vi "TilesLoop.vi"(8 "error in (no error)":errorcluster, 11 "Engine in":refnum<class "Engine.lvclass">) -> (0 "error out":errorcluster)   [LabVIEW 2019, in "RT_Game.lvlib" / "Engine.lvclass"]
uses:
  Engine.lvclass
  TilesLoopData.ctl
  Game/Coordinate.ctl
  Game/SlideJob.ctl
  Game/ScreenSide.ctl
  Engine.lvclass/Engine.ctl
  SetTilesData.ctl
  SetTileData.ctl
  MessageCluster.ctl
  <vilib>/Utility/error.llb/Error Cluster From Error Code.vi
  <vilib>/rvi/errors/niLvFpgaAdjustHostInterfaceError.vi
  Globals.vi
  <vilib>/rvi/interface/nirviMethod/nirviMethod.xnode
  FPGA_Interface.ctl
  FPGA Bitfiles/myriogameconsole_FPGATarget_Main_ntsPRcBZGxk.lvbitx
  Game/Game.lvclass
  <vilib>/FPGAPlugInAG/myRIO-1900/niLvFpga_WriteFifo_myRIO-1900.vi
  <vilib>/rvi/errors/niLvFpgaMergeErrorWithErrorCode.vi
  RT_Game.lvlib
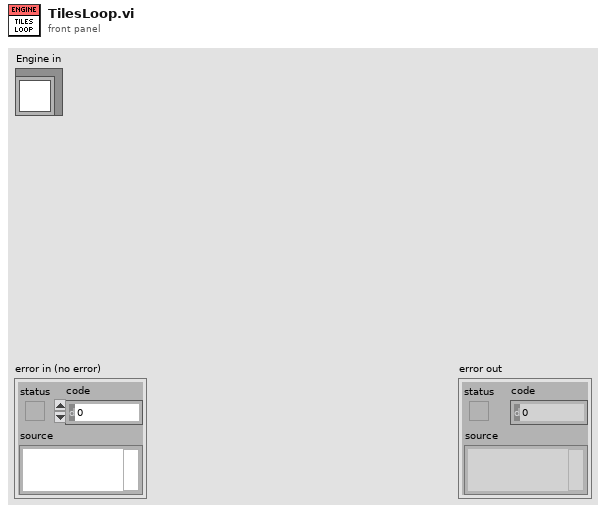
[diagram p1: front panel]
types:
  T1 = typedef "RT_Game.lvlib/Engine.lvclass/TilesLoopData.ctl" = cluster{"TilesToDraw":u64[], "CameraPos":T2, "MoveDistance":T2, "LeftRightBuffer":T3[], "leftrightBufferSize":i16, "leftrightBufferCount":i16, "slidespeed_x":dbl, "delta_t":dbl, "Moving?":bool, "UpDownBuffer":T3[], "updownBufferSize":i16, "updownBufferCount":i16, "slidespeed_y":dbl}
  T2 = typedef "RT_Game.lvlib/Game.lvclass/Coordinate.ctl" = cluster{"x":dbl, "y":dbl}
  T3 = typedef "RT_Game.lvlib/Engine.lvclass/SlideJob.ctl" = cluster{"Pixel":u32[], "Side":T4}
  T4 = typedef "RT_Game.lvlib/Game.lvclass/ScreenSide.ctl" = enum16{"up", "down", "left", "right", "none"}
  T5 = typedef "RT_Game.lvlib/Engine.lvclass/SetTilesData.ctl" = cluster{"TileCodes":u32[][], "Position":T2}
  T6 = typedef "RT_Game.lvlib/Engine.lvclass/SetTileData.ctl" = cluster{"TileCode":u32, "Position":T2}
  T7 = typedef "RT_Game.lvlib/Engine.lvclass/MessageCluster.ctl" = cluster{"Message":string, "Data":variant}
  T8 = typedef "FPGA_Interface.ctl" = refnum<k20>
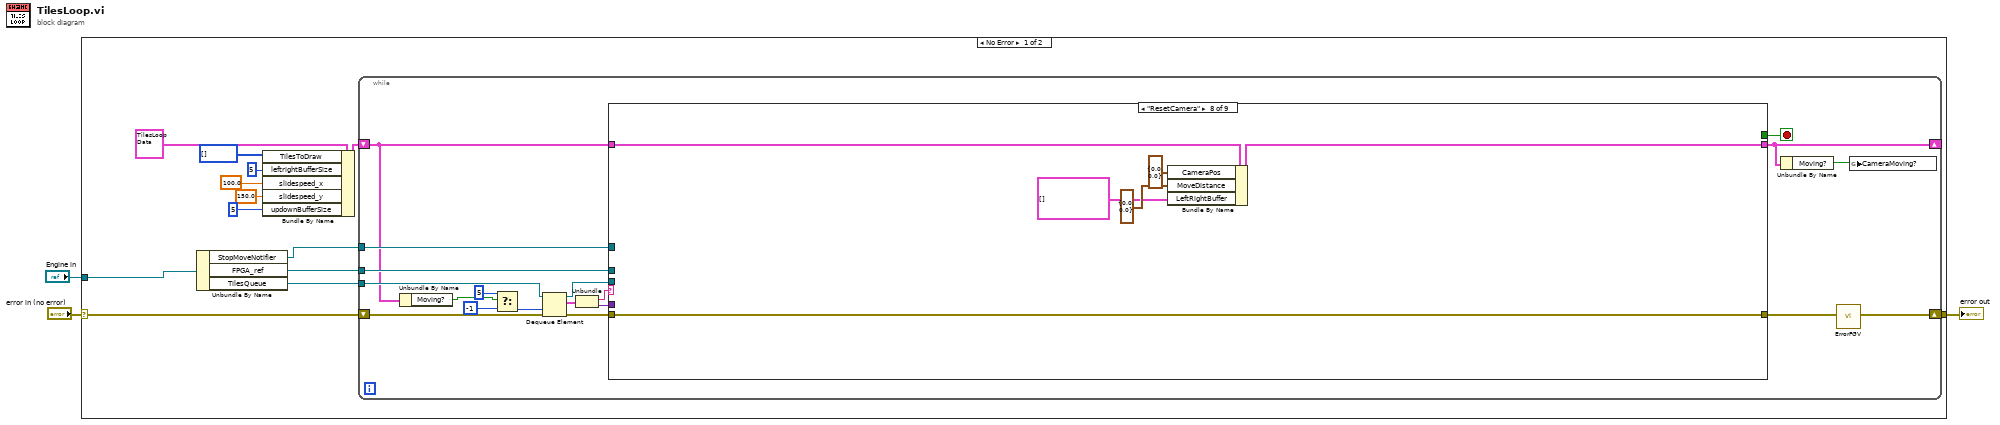
[diagram p0: block diagram]
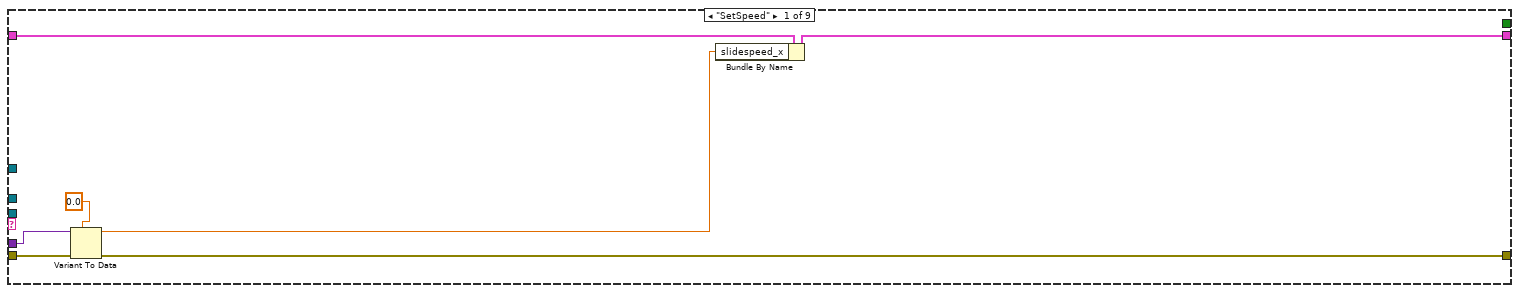
[diagram p2: hidden frame]
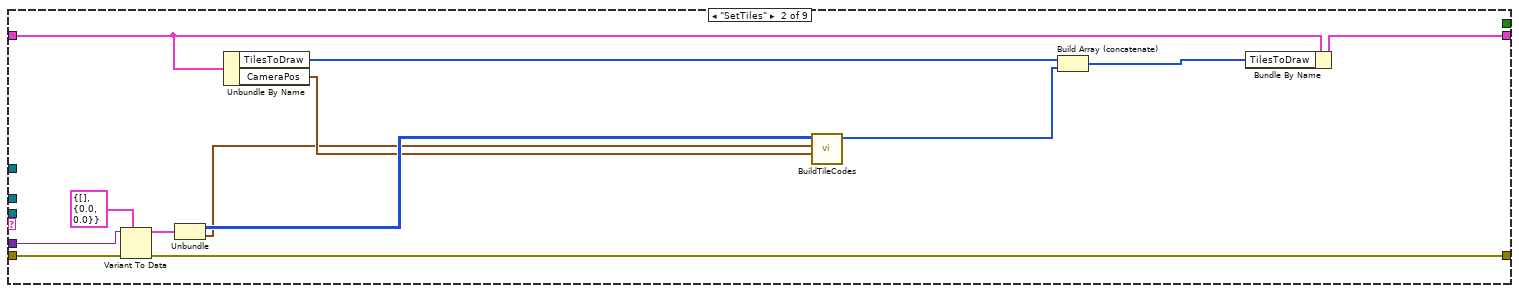
[diagram p3: hidden frame]
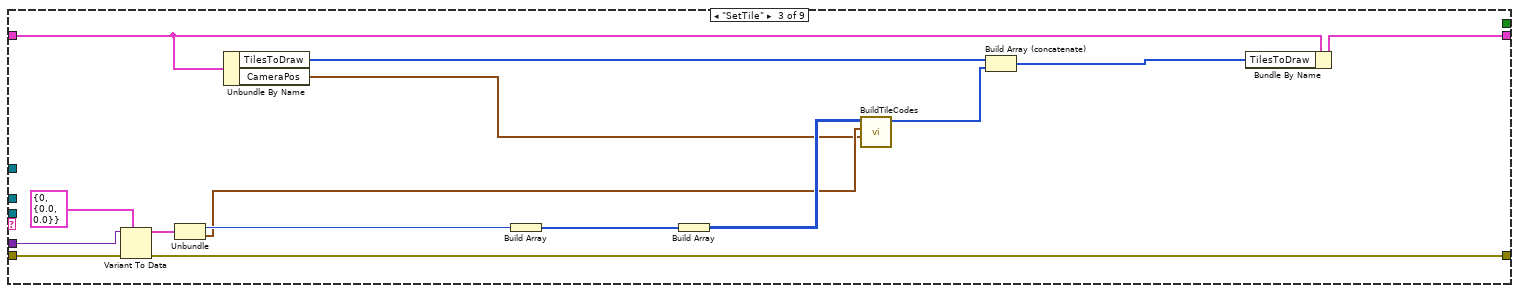
[diagram p4: hidden frame]
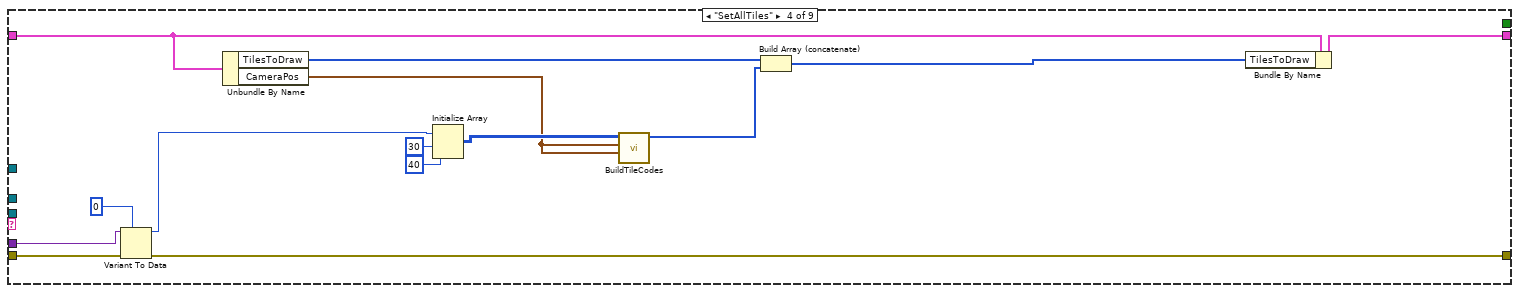
[diagram p5: hidden frame]
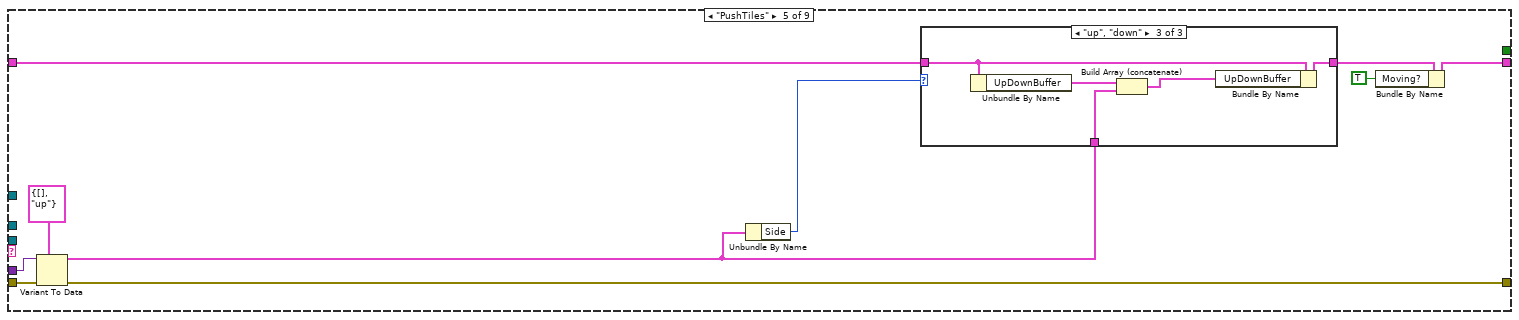
[diagram p6: hidden frame]
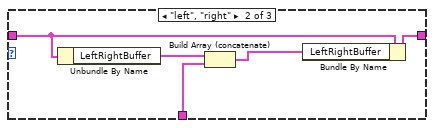
[diagram p8: hidden frame]
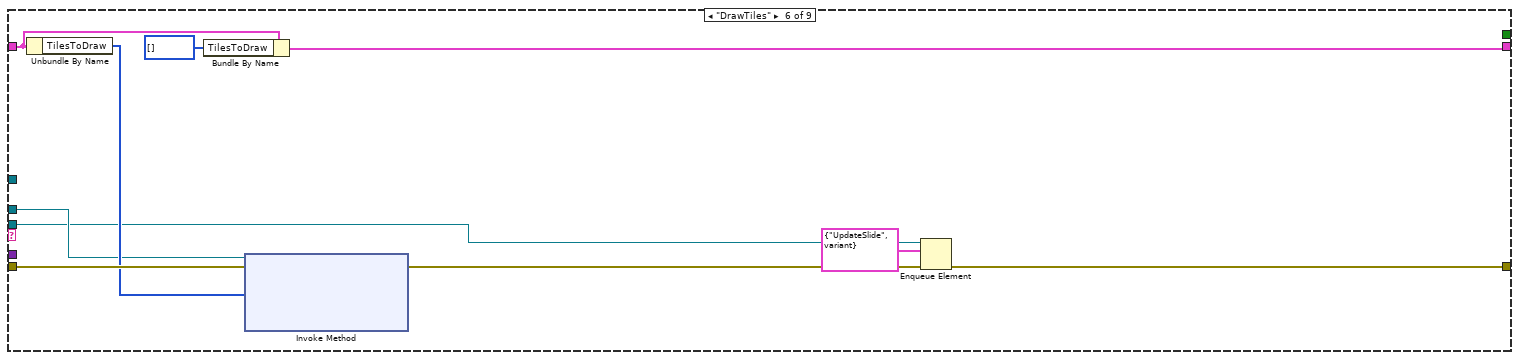
[diagram p9: hidden frame]
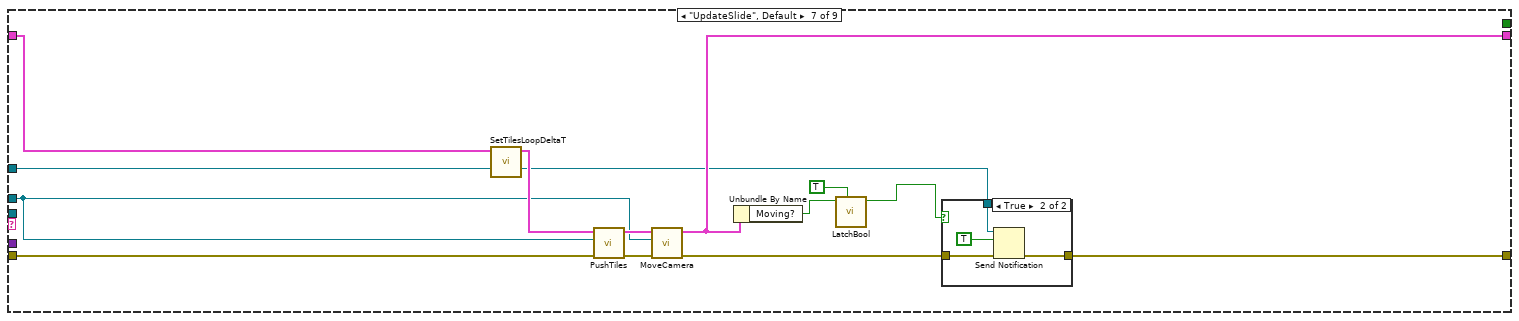
[diagram p10: hidden frame]
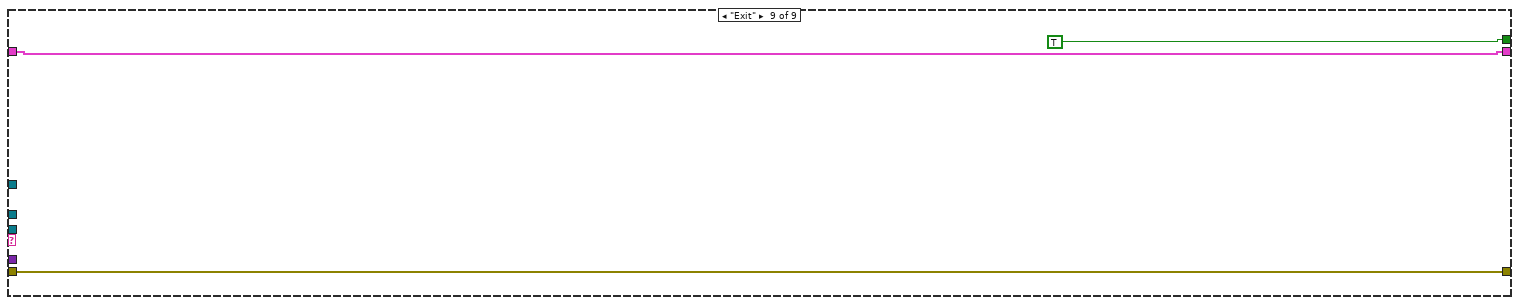
[diagram p12: hidden frame]
diagram:
  n1 = case shown="No Error" "error in (no error)" {
    selector: "error in (no error)" -> [w16 w143]
    tunnel: [w13 w143] -> w2
    tunnel: "Engine in" -> [w15 _]
    frame No Error {
      n2 = Unbundle By Name(w15) -> ("StopMoveNotifier"=w6:refnum<notifier>, "FPGA_ref"=w12:T8, "TilesQueue"=w14:refnum<queue>)
      n3 = Bundle By Name(cluster=T1 {"TilesToDraw"=[], "CameraPos"={"x"=0.0, "y"=0.0}, "MoveDistance"={"x"=0.0, "y"=0.0}, "LeftRightBuffer"=[], "leftrightBufferSize"=0, "leftrightBufferCount"=0, "slidespeed_x"=0.0, "delta_t"=0.0, "Moving?"=FALSE, "UpDownBuffer"=[], "updownBufferSize"=0, "updownBufferCount"=0, "slidespeed_y"=0.0}, "TilesToDraw"=u64[] [], "leftrightBufferSize"=i16 5, "slidespeed_x"=100.0, "slidespeed_y"=150.0 ("delta_t"), "updownBufferSize"=i16 5) -> (w10:T1)
      n4 = while {
        tunnel: w14 -> [w33]
        tunnel: w12 -> [w28]
        shift-right: [w17] -> w13
        shift-left: w16 -> [w35]
        shift-right: [w26] -> _
        shift-left: w10 -> [w21]
        tunnel: w6 -> [w24]
        stop <- w27 stop-if-true
        n5 = Unbundle By Name(w21) -> ("Moving?"=w20:bool)
        n6 = Select(t=5, s=w20, f=-1 ("timeout in ms (-1)")) -> (s? t:f=w22:i32)
        n7 = Dequeue Element(queue=w33, timeout in ms (-1)=w22, error in (no error)=w35) -> (queue out=w18:refnum<queue>, element=w31:T7, error out=w34:errorcluster)  [unwired: 1 out]
        n8 = Unbundle(w31) -> ("Message"=w30:string, "Data"=w29:variant)
        n9 = case shown="\"ResetCamera\"" w30 {
          tunnel: w34 -> [w42 w55 w70 w84 w94 w115 w128 w139 w142]
          tunnel: [w40 w54 w69 w83 w91 w108 w121 w139 w142] -> w32
          tunnel: w29 -> [w39 w53 w68 w82 w90 _ _ _ _]
          tunnel: w28 -> [_ _ _ _ _ w111 w123 _ _]
          tunnel: [_ _ _ _ _ _ _ _ TRUE] -> w27
          tunnel: [w37 w50 w66 w81 w87 w109 w122 w137 w140] -> w26
          tunnel: w21 -> [w41 w49 w65 w80 w92 w112 w116 w138 w140]
          tunnel: w24 -> [_ _ _ _ _ _ w120 _ _]
          tunnel: w18 -> [_ _ _ _ _ w107 _ _ _]
          frame "SetSpeed" {
            n10 = Variant To Data(error in=w42, type=0.0 ("slidespeed_x"), Variant=w39) -> (data=w36:dbl, error out=w40:errorcluster)
            n11 = Bundle By Name(cluster=w41, "slidespeed_x"=w36) -> (w37:T1)
          }
          frame "SetTiles" {
            n12 = Variant To Data(error in=w55, type=T5 {"TileCodes"=[], "Position"={"x"=0.0, "y"=0.0}} ("SetTilesData"), Variant=w53) -> (data=w51:T5, error out=w54:errorcluster)
            n13 = Unbundle(w51) -> ("TileCodes"=w47:u32[][], "Position"=w43:T2)
            n14 = Unbundle By Name(w49) -> ("TilesToDraw"=w48:u64[], "CameraPos"=w44:T2)
            n15 = call "BuildTileCodes.vi"("CameraPos"=w44, "Position"=w43, "TileCodes"=w47) -> ("Array"=w45:u64[])  [unwired: 8 in]
            n16 = Build Array (concatenate)(w48, w45) -> (w46:u64[])
            n17 = Bundle By Name(cluster=w49, "TilesToDraw"=w46) -> (w50:T1)
          }
          frame "SetTile" {
            n18 = Variant To Data(error in=w70, type=T6 {"TileCode"=0, "Position"={"x"=0.0, "y"=0.0}} ("SetTileData"), Variant=w68) -> (data=w67:T6, error out=w69:errorcluster)
            n19 = Unbundle(w67) -> ("TileCode"=w63:u32, "Position"=w60:T2)
            n20 = Unbundle By Name(w65) -> ("TilesToDraw"=w58:u64[], "CameraPos"=w59:T2)
            n21 = Build Array(w63) -> (w62:u32[])
            n22 = Build Array(w62) -> (w61:u32[][])
            n23 = call "BuildTileCodes.vi"("CameraPos"=w59, "Position"=w60, "TileCodes"=w61) -> ("Array"=w56:u64[])  [unwired: 8 in]
            n24 = Build Array (concatenate)(w58, w56) -> (w57:u64[])
            n25 = Bundle By Name(cluster=w65, "TilesToDraw"=w57) -> (w66:T1)
          }
          frame "SetAllTiles" {
            n26 = Variant To Data(error in=w84, type=u32 0 ("TileCode"), Variant=w82) -> (data=w74:u32, error out=w83:errorcluster)
            n27 = Unbundle By Name(w80) -> ("TilesToDraw"=w78:u64[], "CameraPos"=w73:T2)
            n28 = Initialize Array(w74, 30 ("dimension size"), 40 ("dimension size")) -> (w75:u32[][])
            n29 = call "BuildTileCodes.vi"("CameraPos"=w73, "Position"=w73, "TileCodes"=w75) -> ("Array"=w71:u64[])  [unwired: 8 in]
            n30 = Build Array (concatenate)(w78, w71) -> (w72:u64[])
            n31 = Bundle By Name(cluster=w80, "TilesToDraw"=w72) -> (w81:T1)
          }
          frame "PushTiles" {
            n32 = Variant To Data(error in=w94, type=T3 {"Pixel"=[], "Side"=enum."up"} ("SlideJob"), Variant=w90) -> (data=w88:T3, error out=w91:errorcluster)
            n33 = Unbundle By Name(w88) -> ("Side"=w85:T4)
            n34 = case shown="\"up\", \"down\"" w85 {
              tunnel: [w95 w100 w105] -> w93
              tunnel: w92 -> [w95 w99 w104]
              tunnel: w88 -> [_ w96 w101]
              frame Default {
              }
              frame "left", "right" {
                n35 = Unbundle By Name(w99) -> ("LeftRightBuffer"=w98:T3[])
                n36 = Build Array (concatenate)(w98, w96) -> (w97:T3[])
                n37 = Bundle By Name(cluster=w99, "LeftRightBuffer"=w97) -> (w100:T1)
              }
              frame "up", "down" {
                n38 = Unbundle By Name(w104) -> ("UpDownBuffer"=w103:T3[])
                n39 = Build Array (concatenate)(w103, w101) -> (w102:T3[])
                n40 = Bundle By Name(cluster=w104, "UpDownBuffer"=w102) -> (w105:T1)
              }
            }
            n41 = Bundle By Name(cluster=w93, "Moving?"=TRUE) -> (w87:T1)
          }
          frame "DrawTiles" {
            n42 = Unbundle By Name(w112) -> ("TilesToDraw"=w114:u64[])
            n43 = Bundle By Name(cluster=w112, "TilesToDraw"=u64[] []) -> (w109:T1)
            n44 = xnode "Invoke Method"("FPGA VI Reference In"=w111, "error in"=w115, "Data"=w114) -> ("error out"=w110:errorcluster)  [unwired: 1 in, 2 out]
            n45 = Enqueue Element(queue=w107, element=T7 {"Message"="UpdateSlide", "Data"=variant}, error in (no error)=w110) -> (error out=w108:errorcluster)  [unwired: 1 in, 2 out]
          }
          frame "UpdateSlide", Default {
            n46 = call "SetTilesLoopDeltaT.vi"("TilesLoopData in"=w116) -> ("TilesLoopData out"=w126:T1)  [unwired: 10 in]
            n47 = call "PushTiles.vi"("error in (no error)"=w128, "Refnum in"=w123, "TilesLoopData in"=w126) -> ("error out"=w127:errorcluster, "TilesLoopData out"=w124:T1)  [unwired: 7 in]
            n48 = call "MoveCamera.vi"("error in (no error)"=w127, "Refnum in"=w123, "TilesLoopData in"=w124) -> ("error out"=w125:errorcluster, "TilesLoopData out"=w122:T1)  [unwired: 7 in]
            n49 = Unbundle By Name(w122) -> ("Moving?"=w119:bool)
            n50 = call "LatchBool.vi"("falling edge? (f)"=TRUE, "Boolean"=w119) -> ("Latched Boolean"=w118:bool)  [unwired: 9 in]
            n51 = case shown="True" w118 {
              tunnel: w125 -> [w129 w133]
              tunnel: [w129 w132] -> w121
              tunnel: w120 -> [_ w131]
              frame False {
              }
              frame True {
                n52 = Send Notification(notification=TRUE, notifier=w131, error in (no error)=w133) -> (error out=w132:errorcluster)  [unwired: 1 out]
              }
            }
          }
          frame "ResetCamera" {
            n53 = Bundle By Name(cluster=w138, "CameraPos"=T2 {"x"=0.0, "y"=0.0}, "MoveDistance"=T2 {"x"=0.0, "y"=0.0}, "LeftRightBuffer"=T3[] []) -> (w137:T1)
          }
          frame "Exit" {
          }
        }
        n54 = Unbundle By Name(w26) -> ("Moving?"=w25:bool)
        n55 = call "ErrorFGV.vi"("error in (no error)"=w32) -> ("error out"=w17:errorcluster)  [unwired: 9 in, 1 out]
        n56 = global write "Globals.vi" "CameraMoving?"(w25) -> ()
      }
    }
    frame Error {
    }
  }
  "error out" <- w2
